vi "CMN_KeyValToPairs.vi"(9 "replace all? (F)":bool, 10 "key=value pairs":string) -> (2 "arguments out":string)   [LabVIEW 2016]
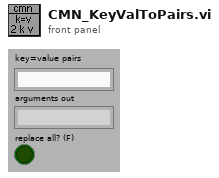
[diagram p1: front panel]
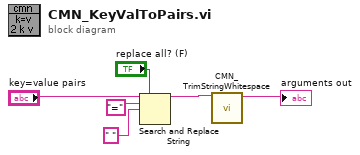
[diagram p0: block diagram]
diagram:
  n1 = Search and Replace String(replace all?="replace all? (F)", input string="key=value pairs", search string="=" ("regular expression"), replace string=" " ("replace string (\"\")")) -> (result string=w3:string)  [unwired: 1 in, 6 out]
  n2 = call "CMN_TrimStringWhitespace.vi"("string"=w3) -> ("trimmed string"=→"arguments out":string)  [unwired: 1 in, 8 out]
